vi "WriteFile.vi"(6 "RefreshTime":u32, 7 "Refnum in":T1, 8 "error in (no error)":errorcluster, 9 "BaseMeasurements":T7 {"NHRGridSim Phase" items=["All", "A Phase", "B Phase", "C Phase"]; "NHRDC Measurement Type" items=["Voltage"=1, "Positive Peak Voltage"=2, "Positive Peak Voltage Last Fetch"=4, "Negative Peak Voltage"=8, "Negative Peak Voltage Last Fetch"=16, "Current"=32, "Positive Peak Current"=64, "Positive Peak Current Last Fetch"=128, "Negative Peak Current"=256, "Negative Peak Current Last Fetch"=512, "Power"=1024, "Positive Peak Power"=2048, "Positive Peak Power Last Fetch"=4096, "Negative Peak Power"=8192, "Negative Peak Power Last Fetch"=16384, "Timestamp"=32768, "Charge Time"=65536, "Discharge Time"=131072, "Amp Hour"=262144, "Amp Hour Time"=524288, "Amp Hour Charge"=1048576, "Amp Hour Discharge"=2097152, "Kilo Watt Hour"=4194304, "Kilo Watt Hour Time"=8388608, "Kilo Watt Hour Charge"=16777216, "Kilo Watt Hour Discharge"=33554432, "UUT Temperature"=67108864]; "NHRDC Fetch Method" items=["Aperture", "Immediate"]}, 10 "BaseConfiguration":T2 {"PPS"."Source Range"."Frequency Range (600Hz)" items=["150 Hz", "300 Hz", "600 Hz", "1200 Hz"]; "PPS"."Source Range"."Range Control (0: Auto)" items=["Auto", "<110 V", "110 V -120.9 V", "121 V - 130.9 V", "> 131 V"]; "PPS"."Program #"."Waveform C (1: Sine)" items=["Sine"=1, "Arbitrary Waveform 2"=2, "Arbitrary Waveform 3"=3, "Arbitrary Waveform 4"=4, "Arbitrary Waveform 5"=5, "Arbitrary Waveform 6"=6, "Arbitrary Waveform 7"=7, "Arbitrary Waveform 8"=8, "Arbitrary Waveform 9"=9, "Arbitrary Waveform 10"=10, "Arbitrary Waveform 11"=11, "Arbitrary Waveform 12"=12, "Arbitrary Waveform 13"=13, "Arbitrary Waveform 14"=14, "Arbitrary Waveform 15"=15, "Arbitrary Waveform 16"=16, "Arbitrary Waveform 17"=17, "Arbitrary Waveform 18"=18, "Arbitrary Waveform 19"=19, "Arbitrary Waveform 20"=20, "Arbitrary Waveform 21"=21, "Arbitrary Waveform 22"=22]; "PPS"."Program #"."Waveform B (1: Sine)" items=["Sine"=1, "Arbitrary Waveform 2"=2, "Arbitrary Waveform 3"=3, "Arbitrary Waveform 4"=4, "Arbitrary Waveform 5"=5, "Arbitrary Waveform 6"=6, "Arbitrary Waveform 7"=7, "Arbitrary Waveform 8"=8, "Arbitrary Waveform 9"=9, "Arbitrary Waveform 10"=10, "Arbitrary Waveform 11"=11, "Arbitrary Waveform 12"=12, "Arbitrary Waveform 13"=13, "Arbitrary Waveform 14"=14, "Arbitrary Waveform 15"=15, "Arbitrary Waveform 16"=16, "Arbitrary Waveform 17"=17, "Arbitrary Waveform 18"=18, "Arbitrary Waveform 19"=19, "Arbitrary Waveform 20"=20, "Arbitrary Waveform 21"=21, "Arbitrary Waveform 22"=22]; "PPS"."Program #"."Coupling  (0: Direct)" items=["Direct", "Transformer"]; "PPS"."Program #"."Form (3: Three)" items=["Single", "Split", "Three"]; "PPS"."Program #"."Program Number (0)" min=1; "PPS"."Program #"."Waveform A (1: Sine)" items=["Sine"=1, "Arbitrary Waveform 2"=2, "Arbitrary Waveform 3"=3, "Arbitrary Waveform 4"=4, "Arbitrary Waveform 5"=5, "Arbitrary Waveform 6"=6, "Arbitrary Waveform 7"=7, "Arbitrary Waveform 8"=8, "Arbitrary Waveform 9"=9, "Arbitrary Waveform 10"=10, "Arbitrary Waveform 11"=11, "Arbitrary Waveform 12"=12, "Arbitrary Waveform 13"=13, "Arbitrary Waveform 14"=14, "Arbitrary Waveform 15"=15, "Arbitrary Waveform 16"=16, "Arbitrary Waveform 17"=17, "Arbitrary Waveform 18"=18, "Arbitrary Waveform 19"=19, "Arbitrary Waveform 20"=20, "Arbitrary Waveform 21"=21, "Arbitrary Waveform 22"=22]; "NHRDC"."OutputSettings"."Wait on Value" items=["Voltage Greater Than Or Equal To", "Voltage Less Than Or Equal To", "Current Greater Than Or Equal To", "Current Less Than Or Equal To", "Power Greater Than Or Equal To", "Power Less Than Or Equal To"]; "NHRDC"."operating state (Off)" items=["Off", "Stand By", "Charge", "Discharge", "Battery Emulation"]; "Chroma"."Phases"."Phase Select" items=["Phase ALL", "Phase A", "Phase B", "Phase C"]}, 11 "ChromaAcLoad in":refnum<class "ChromaAcLoad.lvclass">) -> (0 "error out":errorcluster, 3 "ChromaAcLoad out":refnum<class "ChromaAcLoad.lvclass">)   [LabVIEW 2018, in "AcPwrPlugins.lvlib" / "ChromaAcLoad.lvclass"]
uses:
  ChromaAcLoad.lvclass
  AcPwrBaseClass/AcPwrBase.lvclass
  TypeDefs/DeviceProperties.ctl
  TypeDefs/MeasurementType.ctl
  AcPwrBaseClass/TypeDefs/BaseMeasurements.ctl
  AcPwrBaseClass/TypeDefs/Phase.ctl
  NHRDCPower/TypeDefs/Device(s)Settings.ctl
  NHRDCPower/NHRDCPower.lvclass
  PacificPowerSource/TypeDefs/DeviceSettings.ctl
  PacificPowerSource/PacificPowerSource.lvclass
  AcPwrBaseClass/TypeDefs/BaseConfig.ctl
  <vilib>/Utility/config.llb/Config Data RefNum.ctl
  <vilib>/Utility/config.llb/NI_LVConfig.lvlib
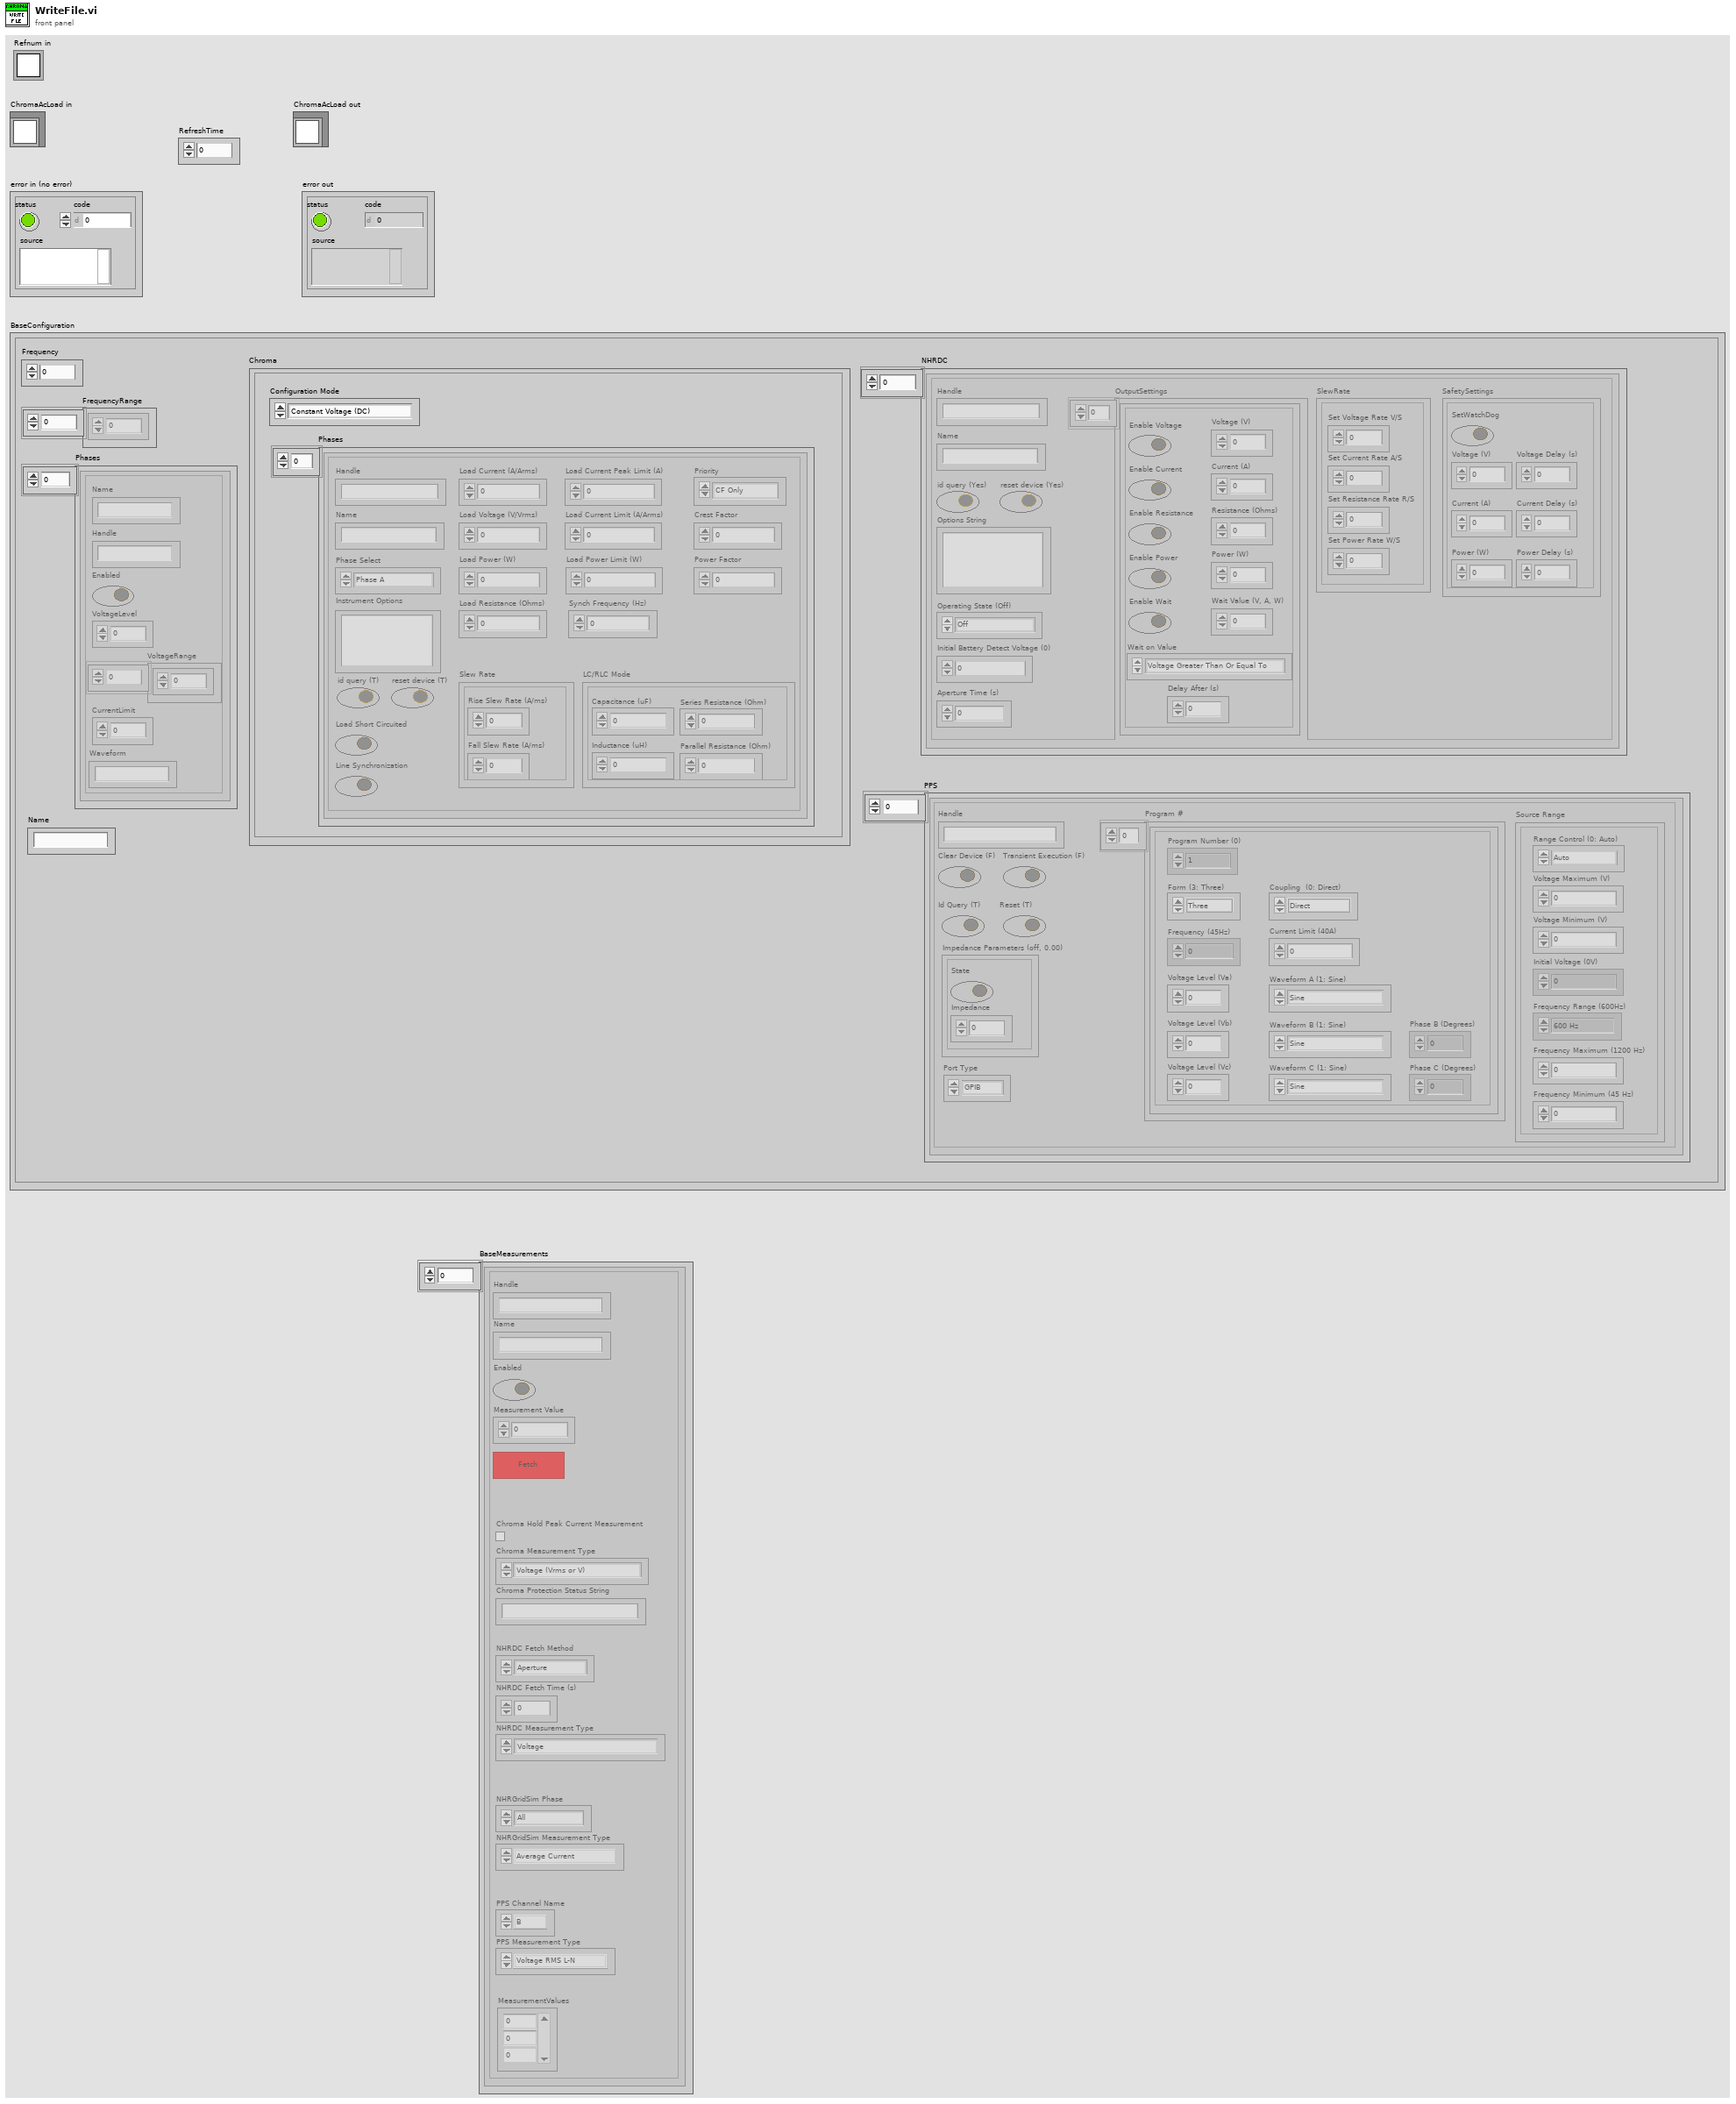
[diagram p1: front panel]
types:
  T1 = typedef "NI_LVConfig.lvlib/Config Data RefNum.ctl" = refnum<k1>
  T2 = typedef "AcPwrPlugins.lvlib/AcPwrBase.lvclass/BaseConfig.ctl" = cluster{"Frequency":dbl, "FrequencyRange":dbl[], "Phases":T3[], "Name":string, "Chroma":T4, "NHRDC":T5, "PPS":T6}
  T3 = typedef "AcPwrPlugins.lvlib/AcPwrBase.lvclass/Phase.ctl" = cluster{"Name":string, "Enabled":bool, "VoltageLevel":dbl, "Handle":string, "VoltageRange":dbl[], "Connected":bool, "CurrentLimit":dbl, "Waveform":string}
  T4 = typedef "AcPwrPlugins.lvlib/ChromaAcLoad.lvclass/DeviceProperties.ctl" = cluster{"Configuration Mode":enum16{"Constant Voltage (DC)", "Constant Power (DC)", "Constant Power (AC)", "Constant Current (DC)", "Constant Current (AC)", "Constant Resistance (DC)", "Constant Resistance (AC)", "Rectified Mode (DC)", "Inrush (AC)", "RLC CP (AC)", "RLC (AC)"}, "Phases":cluster{"Handle":string, "Name":string, "Phase Select":i32, "Instrument Options":string, "id query (T)":bool, "reset device (T)":bool, "Load Short Circuited":bool, "Line Synchronization":bool, "Load Current (A/Arms)":dbl, "Load Voltage (V/Vrms)":dbl, "Load Power (W)":dbl, "Load Resistance (Ohms)":dbl, "Load Current Peak Limit (A)":dbl, "Load Current Limit (A/Arms)":dbl, "Load Power Limit (W)":dbl, "Synch Frequency (Hz)":dbl, "Priority":enum16{"CF Only", "PF Only", "Both (CF)", "Both (PF)"}, "Crest Factor":dbl, "Power Factor":dbl, "Slew Rate":cluster{"Rise Slew Rate (A/ms)":i32, "Fall Slew Rate (A/ms)":i32}, "LC/RLC Mode":cluster{"Capacitance (uF)":i32, "Inductance (uH)":i32, "Series Resistance (Ohm)":dbl, "Parallel Resistance (Ohm)":dbl}, "Timing":cluster{"TimingOn":enum16{""}, "Hours":u32, "Minutes":u32, "Seconds":dbl, "CutoffVoltage":dbl}, "Connected":bool}[]}
  T5 = typedef "AcPwrPlugins.lvlib/NHRDCPower.lvclass/Device(s)Settings.ctl" = cluster{"Handle":string, "Name":string, "id query (Yes)":bool, "reset device (Yes)":bool, "Connected":bool, "Voltage Range (V)":dbl[], "Timing":cluster{"TimingOn":enum16{""}, "Hours":u32, "Minutes":u32, "Seconds":dbl, "CutoffVoltage":dbl}, "Initial Battery Detect Voltage (0)":sgl, "SafetySettings":cluster{"SetWatchDog":bool, "Voltage (V)":sgl, "Current (A)":sgl, "Power (W)":sgl, "Voltage Delay (s)":sgl, "Current Delay (s)":sgl, "Power Delay (s)":sgl}, "Options String":string, "Aperture Time (s)":sgl, "operating state (Off)":i32, "OutputSettings":cluster{"Voltage (V)":sgl, "Current (A)":sgl, "Resistance (Ohms)":sgl, "Power (W)":sgl, "Enable Voltage":bool, "Enable Current":bool, "Enable Resistance":bool, "Enable Power":bool, "Delay After (s)":sgl, "Wait Value (V, A, W)":sgl, "Enable Wait":bool, "Wait on Value":i32}[], "SlewRate":cluster{"Set Voltage Rate V/S":sgl, "Set Current Rate A/S":sgl, "Set Resistance Rate R/S":sgl, "Set Power Rate W/S":sgl}}[]
  T6 = typedef "AcPwrPlugins.lvlib/PacificPowerSource.lvclass/DeviceSettings.ctl" = cluster{"Handle":string, "Connected":bool, "Clear Device (F)":bool, "btnIdQuery":bool, "btnReset":bool, "Program #":cluster{"Phase B (Degrees)":i32, "Waveform A (1: Sine)":i32, "Voltage Level (Va)":dbl, "Program Number (0)":i32, "Voltage Level (Vb) ":dbl, "Form (3: Three)":u16, "Coupling  (0: Direct)":u16, "Frequency (45Hz)":dbl, "Current Limit (40A)":dbl, "Phase C (Degrees)":i32, "Voltage Level (Vc)":dbl, "Waveform B (1: Sine)":i32, "Waveform C (1: Sine)":i32}[], "Impedance Parameters (off, 0.00)":cluster{"State":bool, "Impedance":dbl}, "Transient Execution (F)":bool, "OutputEnabled":bool, "Source Range":cluster{"Frequency Minimum (45 Hz)":dbl, "Frequency Maximum (1200 Hz)":dbl, "Voltage Maximum (V)":dbl, "Voltage Minimum (V)":dbl, "Range Control (0: Auto)":u16, "Initial Voltage (0V)":u16, "Frequency Range (600Hz)":u16}, "Port Type":enum16{"GPIB", "Serial"}}[]
  T7 = typedef "AcPwrPlugins.lvlib/AcPwrBase.lvclass/BaseMeasurements.ctl" = cluster{"Handle":string, "Name":string, "Enabled":bool, "Measurement Value":dbl, "btnMeasFetch":bool, "Chroma Hold Peak Current Measurement":bool, "Chroma Measurement Type":T8, "Chroma Protection Status String":string, "NHRDC Fetch Method":i32, "NHRDC Fetch Time (s)":sgl, "NHRDC Measurement Type":i32, "NHRGridSim Measurement Type ":enum16{"Average Current", "Max Current", "Min Current", "Average Voltage", "Max Voltage", "Min Voltage", "Average True Power", "Max True Power", "Min True Power", "Average Apparent Power", "Max Apparent Power", "Min Apparent Power", "Power Factor", "Crest Factor"}, "NHRGridSim Phase ":i32, "PPS Measurement Type ":enum16{"Voltage RMS L-N", "Voltage RMS L-L", "Frequency", "Current RMS", "Current Peak", "Crest Factor", "Power Factor", "Power VA", "Real Power"}, "PPS Channel Name":enum16{"A", "B", "C"}, "MeasurementValues":dbl[]}[]
  T8 = typedef "AcPwrPlugins.lvlib/ChromaAcLoad.lvclass/MeasurementType.ctl" = enum16{"Voltage (Vrms or V)", "Current (Arms or A)", "Power (W)", "Peak Voltage (V)", "Peak Current (A)", "Peak Power (W)", "Frequency (Hz)", "Resistance (Ohms)", "Voltage Overshoot (V)", "Positive Peak Current (A)", "Voltage Undershoot (V)", "Negative Peak Current (A)", "Apparent Power (VA)", "Reacitive Power (VAR)", "Voltage THD", "Power Factor", "Current's Crest Factor"}
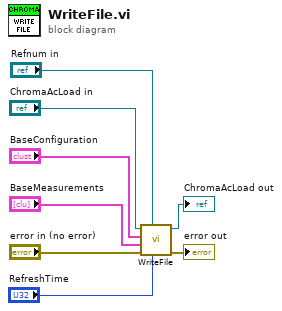
[diagram p0: block diagram]
diagram:
  n1 = call-parent "WriteFile.vi"("RefreshTime"="RefreshTime", "Refnum in"="Refnum in", "error in (no error)"="error in (no error)", "BaseMeasurements"="BaseMeasurements", "BaseConfiguration"="BaseConfiguration", "AcPwrBase in"="ChromaAcLoad in") -> ("error out"=→"error out":errorcluster, "AcPwrBase out"=→"ChromaAcLoad out":refnum<class "ChromaAcLoad.lvclass">)  [unwired: 4 in]
